vi "tempcrtbite.vi"(8 "input":T1, 9 "pulse":u16, 10 "方向":enum8{"正转", "反转\n"}(ring), 11 "ID":enum8{"A", "B"}(ring)) -> (0 "output":T1)   [LabVIEW 2015]
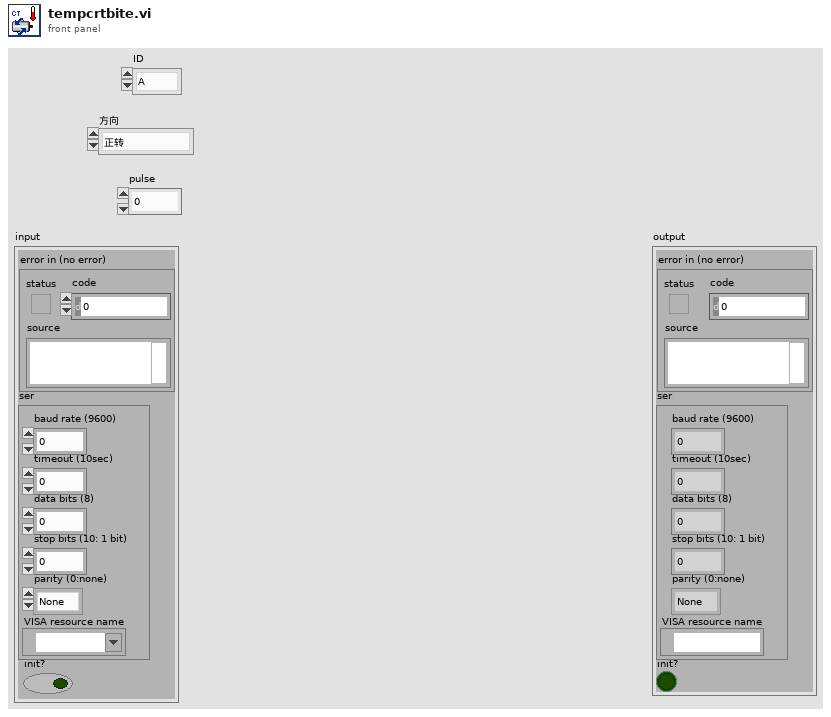
[diagram p1: front panel]
types:
  T1 = cluster{"error in (no error)":errorcluster, "ser":cluster{"baud rate (9600)":u32, "timeout (10sec)":u32, "data bits (8)":u16, "stop bits (10: 1 bit)":u16, "parity (0:none)":enum16{"None", "Odd", "Even", "Mark", "Space"}, "VISA resource name":refnum<visa-resource-name>}, "init?":bool}
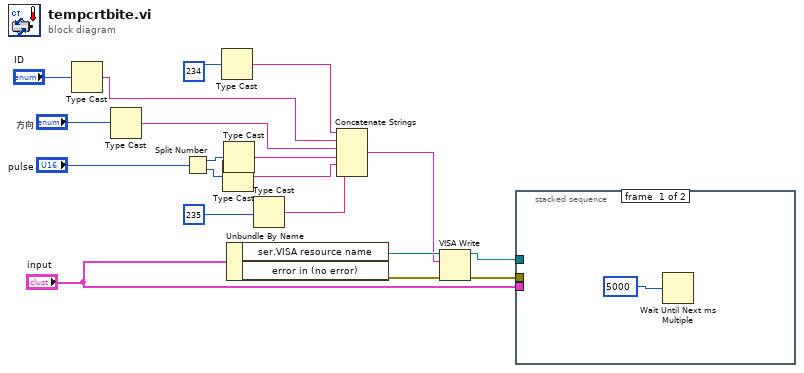
[diagram p0: block diagram]
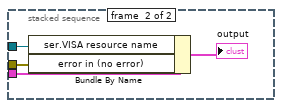
[diagram p2: hidden frame]
diagram:
  n1 = Type Cast(x="ID") -> (*(type *) &x=w3:string)  [unwired: 1 in]
  n2 = Type Cast(x="方向") -> (*(type *) &x=w10:string)  [unwired: 1 in]
  n3 = Split Number(x="pulse") -> (hi(x)=w15:u8, lo(x)=w14:u8)
  n4 = Type Cast(x=u8 234) -> (*(type *) &x=w11:string)  [unwired: 1 in]
  n5 = Type Cast(x=w14) -> (*(type *) &x=w8:string)  [unwired: 1 in]
  n6 = Type Cast(x=w15) -> (*(type *) &x=w9:string)  [unwired: 1 in]
  n7 = Unbundle By Name("input") -> ("ser.VISA resource name"=w18:refnum<visa-resource-name>, "error in (no error)"=w19:errorcluster)
  n8 = Type Cast(x=u8 235) -> (*(type *) &x=w7:string)  [unwired: 1 in]
  n9 = Concatenate Strings(w11, w3, w10, w9, w8, w7) -> (w6:string)
  n10 = VISA Write(VISA resource name=w18, write buffer=w6, error in (no error)=w19) -> (VISA resource name out=w16:refnum<visa-resource-name>, error out=w17:errorcluster)  [unwired: 1 out]
  n11 = stacked-sequence {
    tunnel: w17 -> [_ w24]
    tunnel: w16 -> [_ w23]
    tunnel: "input" -> [_ w22]
    frame #0 {
      n12 = Wait Until Next ms Multiple(millisecond multiple=u32 5000) -> ()  [unwired: 1 out]
    }
    frame #1 {
      n13 = Bundle By Name(cluster=w22, "ser.VISA resource name"=w23, "error in (no error)"=w24) -> (→"output":T1)
    }
  }
